vi "To JSON Tree.vi"(8 "error in (no error)":errorcluster, 11 "error in":refnum<class "error.lvclass">) -> (0 "error out":errorcluster, 2 "JSON out":refnum<class "JSON Null.lvclass">, 3 "error out":refnum<class "error.lvclass">)   [LabVIEW 2015, in "error.lvclass"]
uses:
  error.lvclass
  <vilib>/NI/JSON Support for LabVIEW/JSON Data Classes/JSON Datatype/JSON Null.lvclass
  error.lvclass/error.ctl
  <vilib>/NI/JSON Support for LabVIEW/JSON Data Classes/JSON Object/New JSON Object (Empty).vi
  <vilib>/NI/JSON Support for LabVIEW/JSON Data Classes/JSON Object/Insert Key Value Pair (Single Numeric).vi
  <vilib>/NI/JSON Support for LabVIEW/JSON Data Classes/JSON Object/Insert Key Value Pair (Single String).vi
  <vilib>/NI/JSON Support for LabVIEW/JSON Data Classes/JSON Object/Insert Key Value Pair (Single).vi
  <vilib>/NI/JSON Support for LabVIEW/JSON Data Classes/JSON Helper/JSON Helper.lvclass
  <vilib>/NI/JSON Support for LabVIEW/JSON Data Classes/JSON Object/JSON Object.lvclass
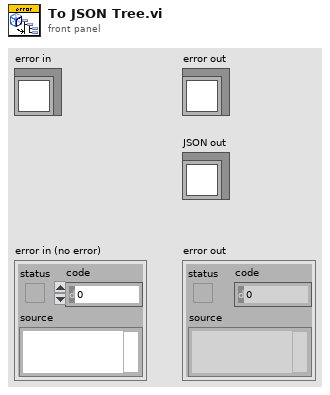
[diagram p1: front panel]
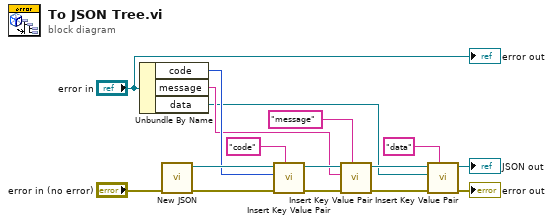
[diagram p0: block diagram]
diagram:
  n1 = Unbundle By Name("error in") -> ("code"=w6:i32, "message"=w5:string, "data"=w4:refnum<class "JSON Null.lvclass">)
  n2 = call-poly <vilib>:"New JSON.vi"("error in (no error)"="error in (no error)") -> ("error out"=w14:errorcluster, "JSON Object out"=w15:refnum<class "JSON Object.lvclass">)  [unwired: 9 in]
  n3 = call-poly <vilib>:"Insert Key Value Pair.vi"("key"="code", "error in (no error)"=w14, "value"=w6, "JSON Object in"=w15) -> ("error out"=w12:errorcluster, "JSON Object out"=w13:refnum<class "JSON Object.lvclass">)  [unwired: 5 in, 1 out]
  n4 = call-poly <vilib>:"Insert Key Value Pair.vi"("key"="message", "error in (no error)"=w12, "value"=w5, "JSON Object in"=w13) -> ("error out"=w10:errorcluster, "JSON Object out"=w11:refnum<class "JSON Object.lvclass">)  [unwired: 5 in, 1 out]
  n5 = call-poly <vilib>:"Insert Key Value Pair.vi"("key"="data", "error in (no error)"=w10, "value"=w4, "JSON Object in"=w11) -> ("error out"=→"error out":errorcluster, "JSON Object out"=→"JSON out":refnum<class "JSON Object.lvclass">)  [unwired: 5 in, 1 out]
  "error out" <- "error in"
